vi "Close GUI.vi"(8 "error in (no error)":errorcluster, 11 "PluginGUI in":refnum<class "PluginGUI.lvclass">) -> (0 "error out":errorcluster, 3 "PluginGUI out":refnum<class "PluginGUI.lvclass">)   [LabVIEW 2020, in "VolatusGUI.lvlib" / "PluginGUI.lvclass"]
uses:
  PluginGUI.lvclass
  PluginGUI.lvclass/PluginGUI.ctl
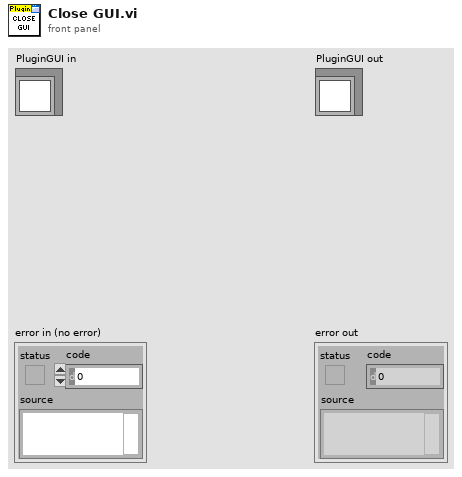
[diagram p1: front panel]
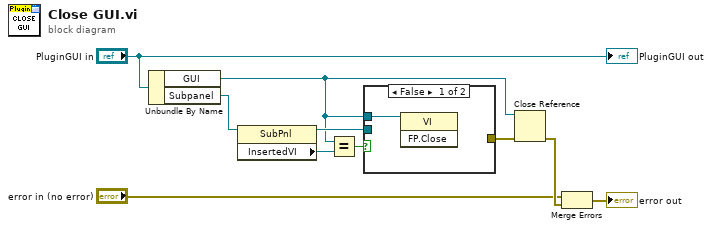
[diagram p0: block diagram]
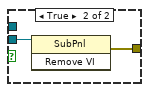
[diagram p2: hidden frame]
diagram:
  n1 = Unbundle By Name("PluginGUI in") -> ("GUI"=w1:refnum<vi>, "Subpanel"=w9:refnum<vi>)
  n2 = property class="SubPnl"(reference=w9) -> (reference out=w6:refnum<vi>, "InsertedVI"=w8:refnum<vi>)  [unwired: 1 in, 1 out]
  n3 = Equal?(x=w1, y=w8) -> (x = y?=w7:bool)
  n4 = case shown="False" w7 {
    tunnel: w6 -> [_ w13]
    tunnel: [_ w12] -> w5
    tunnel: w1 -> [w11 _]
    frame False {
      n5 = invoke class="VI" method="FP.Close"(reference=w11) -> ()  [unwired: 2 in, 3 out]
    }
    frame True {
      n6 = invoke class="SubPnl" method="Remove VI"(reference=w13) -> (error out=w12:errorcluster)  [unwired: 2 in, 2 out]
    }
  }
  n7 = Close Reference(reference=w1, error in (no error)=w5) -> (error out=w4:errorcluster)
  n8 = Merge Errors("error in (no error)", w4) -> (→"error out":errorcluster)
  "PluginGUI out" <- "PluginGUI in"
